vi "test Manage Library.vi"(8 "error in":errorcluster, 11 "test case in":refnum<class "Hardware API.lvclass">) -> (0 "error out":errorcluster, 3 "test case out":refnum<class "Hardware API.lvclass">)   [LabVIEW 2020, in "Hardware API.lvclass"]
uses:
  Hardware API.lvclass
  <vilib>/Analysis/1siggen.llb/Ramp Pattern by Delta.vi
  <vilib>/addons/_JKI Toolkits/VI Tester/TestCase.llb/TestCase.lvclass
  Hardware API/AIM ARINC 429 Hardware API.lvlib
  <vilib>/Analysis/NI_AALBase.lvlib
  C:/Program Files (x86)/National Instruments/LabVIEW 2020/vi.lib/addons/_JKI Toolkits/VI Tester/TestCase.llb/TestCase.lvclass
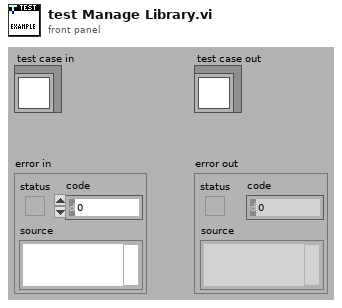
[diagram p1: front panel]
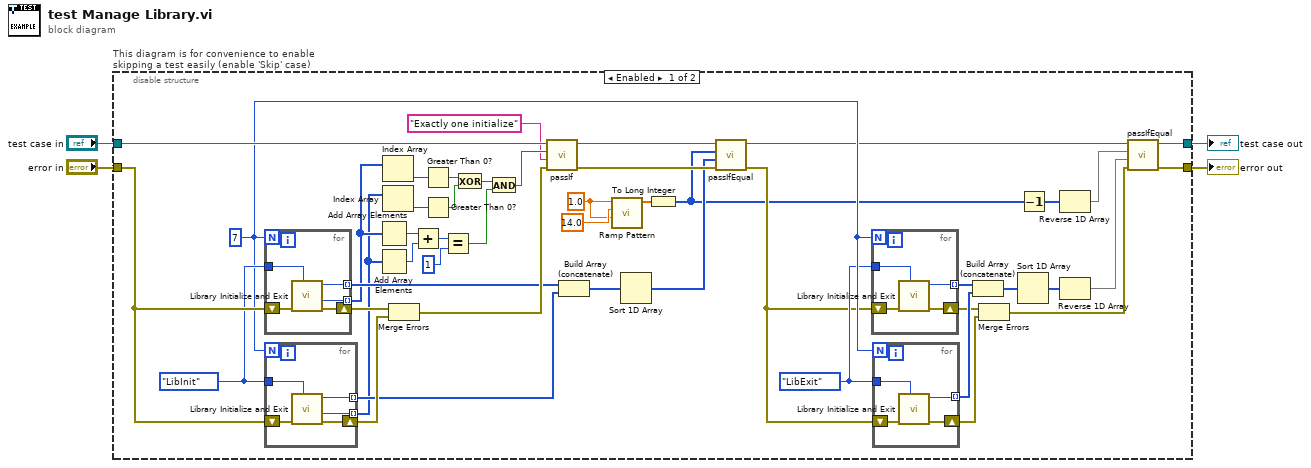
[diagram p0: block diagram]
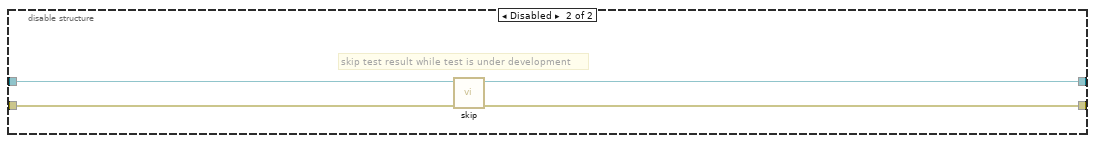
[diagram p2: hidden frame]
diagram:
  n1 = disable-structure "This diagram is for convenience to enable skipping a test easily (enable 'Skip' case)" shown="Enabled" {
    disable-tunnel: "test case in" -> [w50 w72]
    disable-tunnel: [w20 w70] -> w1
    disable-tunnel: [w21 w71] -> w3
    disable-tunnel: "error in" -> [w47 w69]
    frame Enabled {
      w34 = enum16{"LibInit", "LibExit"}."LibExit" ("action")
      w36 = enum16{"LibInit", "LibExit"}."LibInit" ("action")
      w38 = 1.0 ("delta")
      w35 = 7
      n2 = for {
        N: w35 -> [_]
        shift-right: [w67] -> w49
        shift-left: w47 -> [w68]
        tunnel: [w66] -> w14 mode=indexing
        tunnel: [w65] -> w45 mode=indexing
        tunnel: w36 -> [w64]
        n3 = call "Library Initialize and Exit.vi"("action"=w64, "error in"=w68) -> ("error out"=w67:errorcluster, "modules found"=w66:i32, "instance count"=w65:i32)  [unwired: 7 in]
      }
      n4 = for {
        N: w35 -> [_]
        shift-right: [w62] -> w48
        shift-left: w47 -> [w63]
        tunnel: [w61] -> w13 mode=indexing
        tunnel: [w60] -> w44 mode=indexing
        tunnel: w36 -> [w59]
        n5 = call "Library Initialize and Exit.vi"("action"=w59, "error in"=w63) -> ("error out"=w62:errorcluster, "modules found"=w61:i32, "instance count"=w60:i32)  [unwired: 7 in]
      }
      n6 = Add Array Elements(numeric array=w14) -> (sum=w12:i32)
      n7 = Add Array Elements(numeric array=w13) -> (sum=w11:i32)
      n8 = Index Array(array=w14) -> (element=w17:i32)  [unwired: 1 in]
      n9 = Index Array(array=w13) -> (element=w18:i32)  [unwired: 1 in]
      n10 = Merge Errors(w49, w48) -> (w46:errorcluster)
      n11 = Add(x=w12, y=w11) -> (x+y=w10:i32)
      n12 = Greater Than 0?(x=w17) -> (x > 0?=w16:bool)
      n13 = Greater Than 0?(x=w18) -> (x > 0?=w15:bool)
      n14 = Equal?(x=w10, y=1) -> (x = y?=w7:bool)
      n15 = Exclusive Or(1:w15, 2:w16) -> (0:w8:bool)
      n16 = And(x=w8, y=w7) -> (x .and. y?=w6:bool)
      n17 = call-dynamic "passIf.vi"("error in (no error)"=w46, "message (\"\")"="Exactly one initialize" ("message (\"\")"), "pass"=w6, "TestCase in"=w50) -> ("error out"=w41:errorcluster, "TestCase out"=w42:refnum<class "Hardware API.lvclass">)  [unwired: 6 in]
      n18 = Build Array (concatenate)(w45, w44) -> (w43:i32[])
      n19 = call-poly <vilib>:"Ramp Pattern.vi"("start"=w38, "end"=14.0, "delta"=w38) -> ("Ramp Pattern"=w37:dbl[])  [unwired: 6 in, 2 out]
      n20 = Sort 1D Array(array=w43) -> (sorted array=w40:i32[])
      n21 = To Long Integer(number=w37) -> (32bit integer=w28:i32[])
      n22 = call-dynamic "passIfEqual.vi"("error in (no error)"=w41, "y"=w40, "x"=w28, "TestCase in"=w42) -> ("error out"=w33:errorcluster, "TestCase out"=w27:refnum<class "Hardware API.lvclass">)  [unwired: 6 in]
      n23 = for {
        N: w35 -> [_]
        shift-right: [w57] -> w26
        shift-left: w33 -> [w58]
        tunnel: [w56] -> w32 mode=indexing
        tunnel: w34 -> [w55]
        n24 = call "Library Initialize and Exit.vi"("action"=w55, "error in"=w58) -> ("error out"=w57:errorcluster, "instance count"=w56:i32)  [unwired: 7 in, 1 out]
      }
      n25 = for {
        N: w35 -> [_]
        shift-right: [w53] -> w25
        shift-left: w33 -> [w54]
        tunnel: [w52] -> w31 mode=indexing
        tunnel: w34 -> [w51]
        n26 = call "Library Initialize and Exit.vi"("action"=w51, "error in"=w54) -> ("error out"=w53:errorcluster, "instance count"=w52:i32)  [unwired: 7 in, 1 out]
      }
      n27 = Build Array (concatenate)(w32, w31) -> (w30:i32[])
      n28 = Merge Errors(w26, w25) -> (w22:errorcluster)
      n29 = Sort 1D Array(array=w30) -> (sorted array=w29:i32[])
      n30 = Decrement(x=w28) -> (x-1=w19:i32[])
      n31 = Reverse 1D Array(array=w19) -> (reversed array=w24:i32[])
      n32 = Reverse 1D Array(array=w29) -> (reversed array=w23:i32[])
      n33 = call-dynamic "passIfEqual.vi"("error in (no error)"=w22, "y"=w23, "x"=w24, "TestCase in"=w27) -> ("error out"=w21:errorcluster, "TestCase out"=w20:refnum<class "Hardware API.lvclass">)  [unwired: 6 in]
    }
    frame Disabled {
      # "skip test result while test is under development"
      n34 = call <vilib>:"skip.vi"("error in (no error)"=w69, "TestCase in"=w72) -> ("error out"=w71:errorcluster, "TestCase out"=w70:refnum<class "Hardware API.lvclass">)  [unwired: 8 in]
    }
  }
  "error out" <- w3
  "test case out" <- w1
